vi "Write Sub Panel.vi"(8 "error in (no error)":errorcluster, 10 "Sub Panel":refnum<vi>, 11 "Sub Panel Actor in":refnum<class "Sub Panel Actor.lvclass">) -> (0 "error out":errorcluster, 3 "Sub Panel Actor out":refnum<class "Sub Panel Actor.lvclass">)   [LabVIEW 2020, in "Sub Panel Actor.lvlib" / "Sub Panel Actor.lvclass"]
uses:
  Sub Panel Actor.lvclass
  Sub Panel Actor.lvclass/Sub Panel Actor.ctl
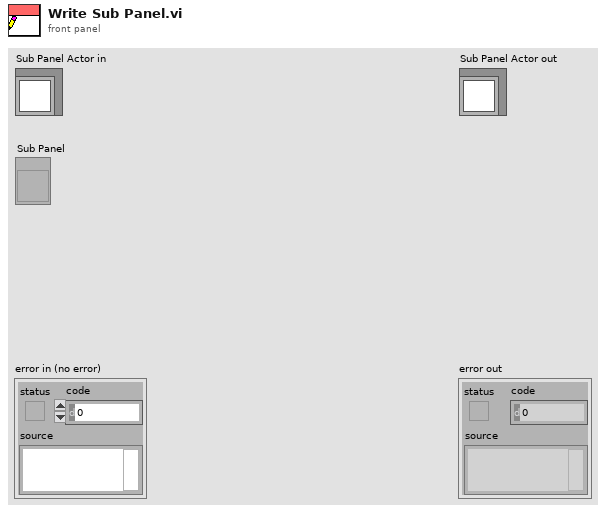
[diagram p1: front panel]
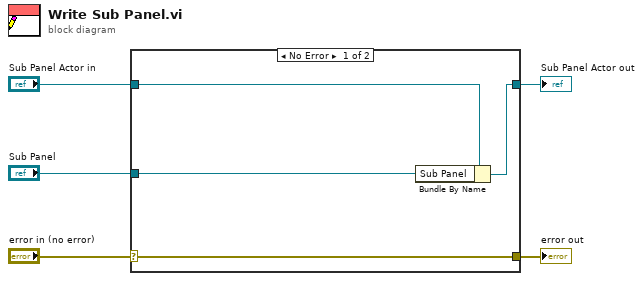
[diagram p0: block diagram]
diagram:
  n1 = case shown="No Error" "error in (no error)" {
    selector: "error in (no error)" -> [w9 w10]
    tunnel: [w9 w10] -> w4
    tunnel: [w7 w11] -> w2
    tunnel: "Sub Panel Actor in" -> [w8 w11]
    tunnel: "Sub Panel" -> [w6 _]
    frame No Error {
      n2 = Bundle By Name(cluster=w8, "Sub Panel"=w6) -> (w7:refnum<class "Sub Panel Actor.lvclass">)
    }
    frame Error {
    }
  }
  "error out" <- w4
  "Sub Panel Actor out" <- w2
